vi "Initalize.vi"(8 "error in (no error)":errorcluster, 11 "Door Actuator in":refnum<class "Door Actuator.lvclass">) -> (0 "error out":errorcluster, 3 "Door Actuator out":refnum<class "Door Actuator.lvclass">)   [LabVIEW 2020, in "Door Actuator.lvclass"]
uses:
  Door Actuator.lvclass
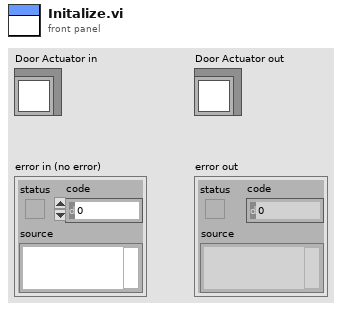
[diagram p1: front panel]
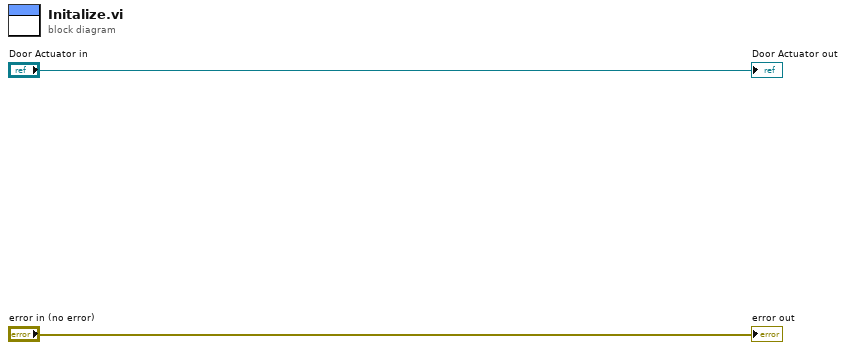
[diagram p0: block diagram]
diagram:
  "error out" <- "error in (no error)"
  "Door Actuator out" <- "Door Actuator in"
